vi "splitting analysis.vi"() -> ()   [LabVIEW 2013]
uses:
  <vilib>/Utility/miscctls.llb/LVOffsetAndMultiplierTypeDef.ctl
panel:
  in  "single file?":bool=TRUE
  in  "Write ITX?":bool
  in  "length":i32=200
  in  "saved ITX":path=path "P:/expt/IQC/2011-summer Superconductivity-Spin Hall/Data/SA02701G.20140330/Processed Data/T dependence analysis"
  in  "filename":string="SA02701G"
  in  "String":string="SA02701G.20140330\nVbg=-0.7 V\nassume coupling factor 0.048\n2nd peak splitting at Vsg=-92 mV"
  out "g factor":cluster{dbl[], dbl[]}[](graph)=[{[200.0, 300.0, 400.0, 500.0, 600.0, 700.0, 800.0, 900.0], [0.762950852924121, 0.7566109708678899, 0.7793059646834901, 0.8038354742392615, 0.847781234879375, 0.95800866075335, 1.1121861322275977, 2.1069962193585083]}, {[200.0, 300.0, 400.0, 500.0, 600.0, 700.0, 800.0, 900.0], [0.9904700666991226, 0.7593959833590997, 0.7931872725452133, 0.8096951324286941, 0.8484508177839173, 0.9257931178365144, 1.0883960545328897, 1.8645473393227352]}]
  in  "stop":bool
  out "Bc":cluster{dbl[], dbl[]}[](graph)=[{[200.0, 300.0, 400.0, 500.0, 600.0, 700.0, 800.0, 900.0], [18681.74837307599, 17246.39341842541, 19078.384544421766, 21540.781211196714, 25094.74708402069, 29025.148908008065, 35530.24026512017, 46884.043989967184]}, {[200.0, 300.0, 400.0, 500.0, 600.0, 700.0, 800.0, 900.0], [35439.925521611505, 23043.21538990028, 24829.07547221065, 26913.878099501664, 29857.458001018036, 33669.416498994, 39732.163472639135, 50971.08969607113]}]
  in  "X Scale":T1={"Offset"=-0.1, "Multiplier"=7.5e-05}
  in  "T":dbl[](array[numeric])=[200.0, 300.0, 400.0, 500.0, 600.0, 700.0, 800.0, 900.0] format="%#_13g"
  in  "regular expression":string="mK"
  in  "data":path=path "P:/expt/IQC/2011-summer Superconductivity-Spin Hall/Data/SA02701J.20140327/sweepVsg-lockin_base_appliedVsd350.000u"
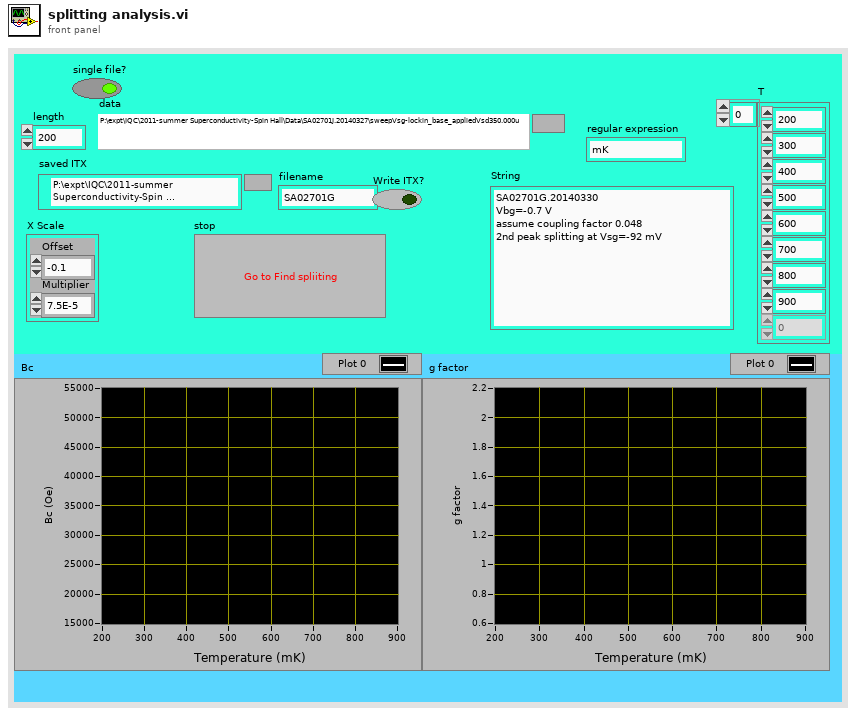
[diagram p1: front panel]
types:
  T1 = typedef "LVOffsetAndMultiplierTypeDef.ctl" = cluster{"Offset":dbl, "Multiplier":dbl}
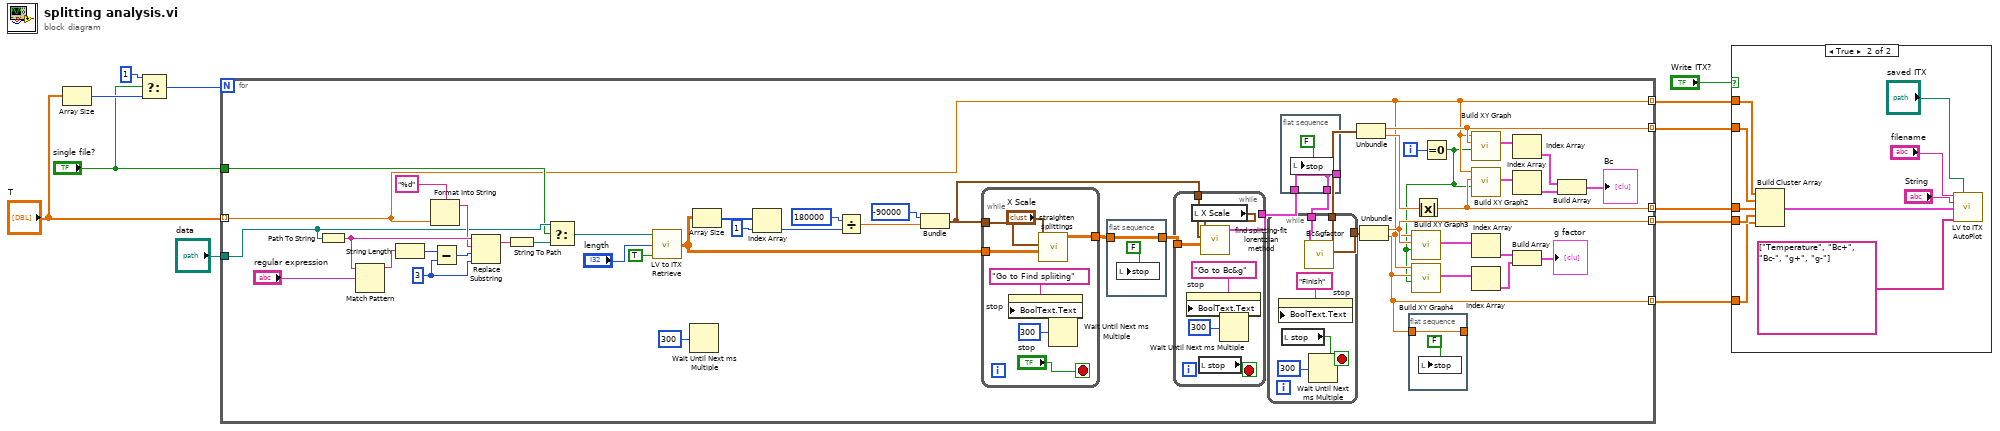
[diagram p0: block diagram]
diagram:
  n1 = Array Size(array="T") -> (size(s)=w4:i32)
  n2 = Select(t=1, s="single file?", f=w4) -> (s? t:f=w3:i32)
  n3 = for {
    N: w3 -> [_]
    tunnel: "data" -> [w37]
    tunnel: "T" -> [w24] mode=indexing
    tunnel: [w34] -> w10 mode=indexing
    tunnel: [w33] -> w9 mode=indexing
    tunnel: [w24] -> w11 mode=indexing
    tunnel: [w26] -> w8 mode=indexing
    tunnel: [w15] -> w7 mode=indexing
    tunnel: "single file?" -> [w35]
    i -> [w27]
    w56 = 3 ("length (len. of substring)")
    n4 = Path To String(path=w37) -> (string=w58:string)
    n5 = Match Pattern(string=w58, regular expression="regular expression") -> (before substring=w59:string)  [unwired: 1 in, 3 out]
    n6 = String Length(string=w59) -> (length=w57:i32)
    n7 = Format Into String(format string="%d", w24) -> (resulting string=w53:string)  [unwired: 2 in, 1 out]
    n8 = Subtract(x=w57, y=w56) -> (x-y=w55:i32)
    n9 = Replace Substring(2:w56, 3:w55, 4:w53, 5:w58) -> (1:w52:string)  [unwired: 1 out]
    n10 = String To Path(string=w52) -> (path=w38:path)
    n11 = Select(t=w37, s=w35, f=w38) -> (s? t:f=w36:path)
    n12 = call <userlib>:"LV to ITX  Retrieve.vi"("File or Folder Path"=w36, "length"="length", "stop"=TRUE) -> ("E"=w50:dbl[][])  [unwired: 8 in, 4 out]
    n13 = Wait Until Next ms Multiple(millisecond multiple=u32 300) -> ()  [unwired: 1 out]
    n14 = Array Size(array=w50) -> (size(s)=w49:i32[])
    n15 = Index Array(array=w49, index=1) -> (element=w45:i32)
    n16 = Divide(x=180000 ("length (len. of substring)"), y=w45) -> (x/y=w44:dbl)
    n17 = Bundle("length (len. of substring)"=-90000, w44) -> (w43:cluster{"length (len. of substring)":i32, dbl})  [unwired: 1 in]
    n18 = while {
      tunnel: w50 -> [w86]
      tunnel: w43 -> [w85]
      tunnel: [w84] -> w19
      stop <- "stop" stop-if-true
      n19 = property on="stop" class="Bool (strict)"("BoolText.Text"="Go to Find spliiting" ("Boolean Text.Text")) -> ()  [unwired: 2 in, 2 out]
      n20 = call "straighten splittings.vi"("E"=w86, "Y Scale.Offset and Multiplier"=w85, "X Scale.Offset and Multiplier"="X Scale") -> ("E 2"=w84:dbl[][])  [unwired: 8 in]
      n21 = Wait Until Next ms Multiple(millisecond multiple=u32 300) -> ()  [unwired: 1 out]
    }
    n22 = flat-sequence {
      tunnel: w19 -> [w78]
      tunnel: [w78] -> w18
      frame #0 {
        n23 = local write "stop"(FALSE ("stop")) -> ()
      }
    }
    n24 = while {
      tunnel: w43 -> [w77]
      tunnel: [w76] -> w17
      tunnel: w18 -> [w75]
      stop <- w73 stop-if-true
      n25 = property on="stop" class="Bool (strict)"("BoolText.Text"="Go to Bc&g" ("Boolean Text.Text")) -> ()  [unwired: 2 in, 2 out]
      n26 = local read "X Scale"() -> (w72:T1)
      n27 = local read "stop"() -> (w73:bool)
      n28 = call "find splitting-fit lorentzian method.vi"("E"=w75, "Y Scale"=w77, "X Scale"=w72) -> ("XY Graph 4"=w76:cluster{dbl[], dbl[]}[])  [unwired: 8 in]
      n29 = Wait Until Next ms Multiple(millisecond multiple=u32 300) -> ()  [unwired: 1 out]
    }
    n30 = while {
      tunnel: [w68] -> w42
      tunnel: [w67] -> w39
      tunnel: w16 -> [w66]
      stop <- w64 stop-if-true
      n31 = property on="stop" class="Bool (strict)"("BoolText.Text"="Finish" ("Boolean Text.Text")) -> ()  [unwired: 2 in, 2 out]
      n32 = local read "stop"() -> (w64:bool)
      n33 = call "Bc&gfactor.vi"("XY Graph 4"=w66) -> ("g factor"=w67:cluster{"g+":dbl, "g-":dbl}, "Bc"=w68:cluster{"Bc+":dbl, "Bc-":dbl})  [unwired: 9 in]
      n34 = Wait Until Next ms Multiple(millisecond multiple=u32 300) -> ()  [unwired: 1 out]
    }
    n35 = flat-sequence {
      tunnel: [w69] -> _
      tunnel: w17 -> [w69]
      tunnel: [w69] -> w16
      frame #0 {
        n36 = local write "stop"(FALSE ("stop")) -> ()
      }
    }
    n37 = Unbundle(w42) -> ("Bc+"=w34:dbl, "Bc-"=w41:dbl)
    n38 = Unbundle(w39) -> ("g+"=w26:dbl, "g-"=w15:dbl)
    n39 = flat-sequence {
      tunnel: w15 -> [w61]
      tunnel: [w61] -> _
      frame #0 {
        n40 = local write "stop"(FALSE ("stop")) -> ()
      }
    }
    n41 = Absolute Value(x=w41) -> (abs(x)=w33:dbl)
    n42 = Equal To 0?(x=w27) -> (x = 0?=w14:bool)
    n43 = call "Build XY Graph3"("Reset"=w14, "Y Input"=w26, "X Input"=w24) -> ("XY Graph"=w25:cluster{"X":dbl[], "Y":dbl[]}[])  [unwired: 7 in, 1 out]
    n44 = call "Build XY Graph4"("Reset"=w14, "Y Input"=w15, "X Input"=w24) -> ("XY Graph"=w23:cluster{"X":dbl[], "Y":dbl[]}[])  [unwired: 7 in, 1 out]
    n45 = call "Build XY Graph"("Reset"=w14, "Y Input"=w34, "X Input"=w24) -> ("XY Graph"=w32:cluster{"X":dbl[], "Y":dbl[]}[])  [unwired: 7 in, 1 out]
    n46 = call "Build XY Graph2"("Reset"=w14, "Y Input"=w33, "X Input"=w24) -> ("XY Graph"=w31:cluster{"X":dbl[], "Y":dbl[]}[])  [unwired: 7 in, 1 out]
    n47 = Index Array(array=w25) -> (element=w21:cluster{"X":dbl[], "Y":dbl[]})  [unwired: 1 in]
    n48 = Index Array(array=w23) -> (element=w22:cluster{"X":dbl[], "Y":dbl[]})  [unwired: 1 in]
    n49 = Index Array(array=w32) -> (element=w30:cluster{"X":dbl[], "Y":dbl[]})  [unwired: 1 in]
    n50 = Index Array(array=w31) -> (element=w29:cluster{"X":dbl[], "Y":dbl[]})  [unwired: 1 in]
    n51 = Build Array(w21, w22) -> (→"g factor":cluster{"X":dbl[], "Y":dbl[]}[])
    n52 = Build Array(w30, w29) -> (→"Bc":cluster{"X":dbl[], "Y":dbl[]}[])
  }
  n53 = case shown="True" "Write ITX?" {
    tunnel: w11 -> [_ w96]
    tunnel: w10 -> [_ w95]
    tunnel: w9 -> [_ w94]
    tunnel: w8 -> [_ w93]
    tunnel: w7 -> [_ w92]
    frame False {
    }
    frame True {
      n54 = Build Cluster Array(w96, w95, w94, w93, w92) -> (w91:cluster{dbl[]}[])
      n55 = call <userlib>:"LV to ITX AutoPlot.vi"("filename"="filename", "path"="saved ITX", "Notes"="String", "Data"=w91, "wavenames (.Vx, etc)"=string[] ["Temperature", "Bc+", "Bc-", "g+", "g-"]) -> ()  [unwired: 10 in, 1 out]
    }
  }
